vi "Data Initialize.vi"(6 "Initialize":bool, 9 "Compensation in":dbl[](array[numeric]), 10 "Data in":dbl[](array[numeric]), 11 "Set Data":dbl[](array[numeric])) -> (2 "Data out":dbl[](array[numeric]), 3 "Compensation out":dbl[](array[numeric]))   [LabVIEW 2021]
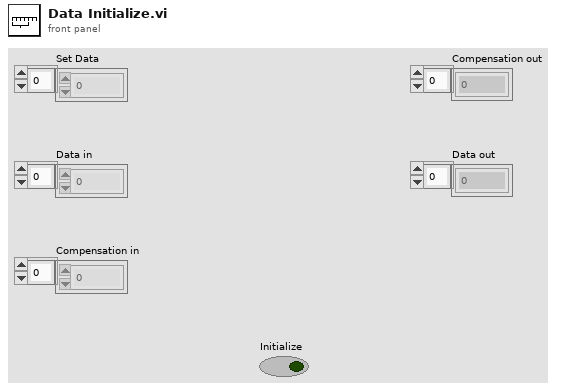
[diagram p1: front panel]
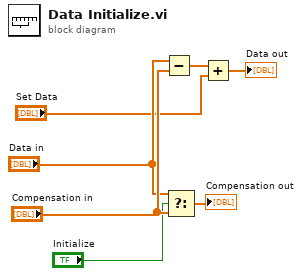
[diagram p0: block diagram]
diagram:
  n1 = Subtract(x="Data in", y="Compensation in") -> (x-y=w2:dbl[])
  n2 = Select(t="Data in", s="Initialize", f="Compensation in") -> (s? t:f=→"Compensation out":dbl[])
  n3 = Add(x=w2, y="Set Data") -> (x+y=→"Data out":dbl[])
